vi "TuningPanel.vi"() -> ()   [LabVIEW 2014]
panel:
  in  "Cancel Button":bool
  in  "TCPConRef":refnum<k5>
  in  "Tuning Element":u16(ring) items=["NonlinearPID", "KalmanFilterRegular", "KalmanFilterAltitude", "AttitudeObserver", "HGObserver"]
  in  "OK Button":bool
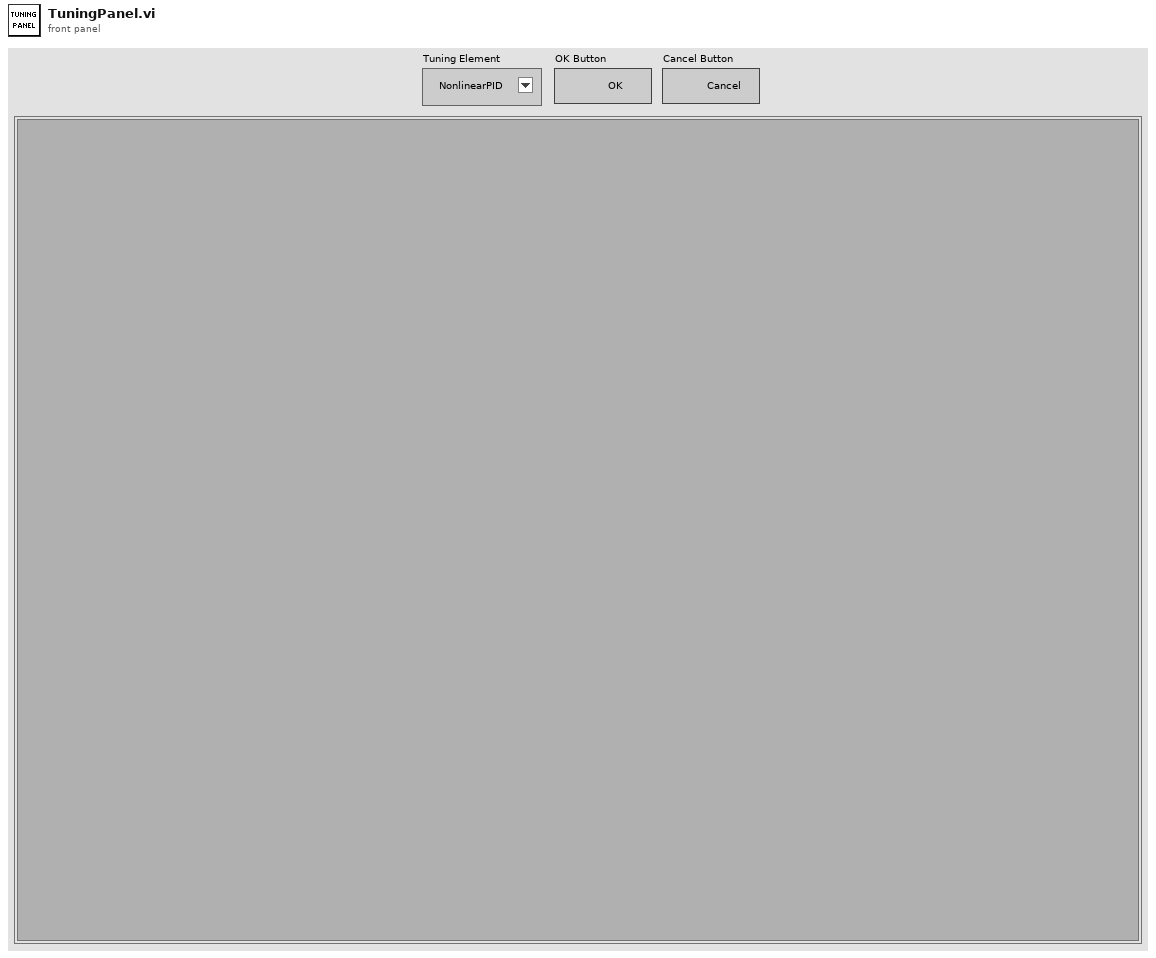
[diagram p1: front panel]
types:
  T1 = enum16{"open", "replace", "create", "open or create", "replace or create", "replace or create with confirmation"}
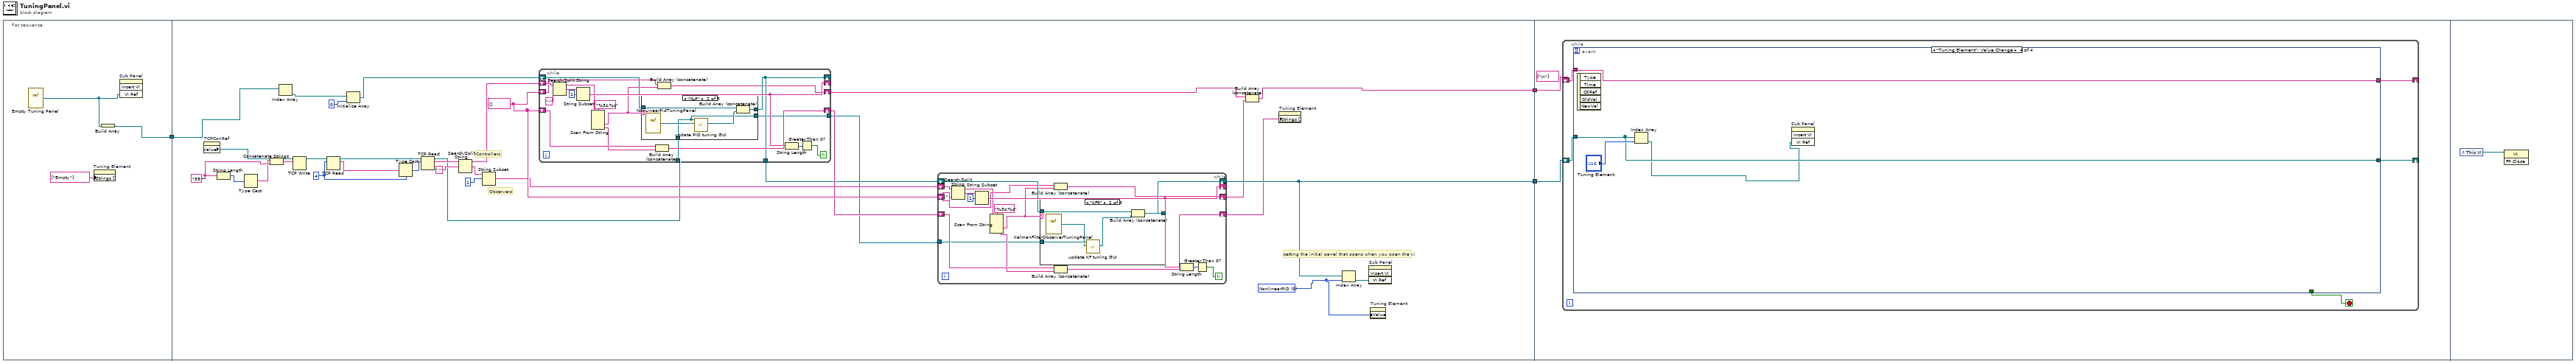
[diagram p0: block diagram]
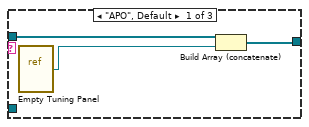
[diagram p2: hidden frame]
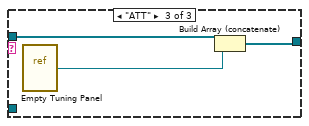
[diagram p3: hidden frame]
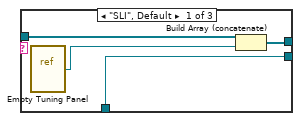
[diagram p4: hidden frame]
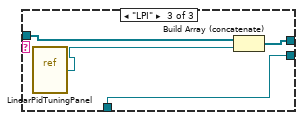
[diagram p5: hidden frame]
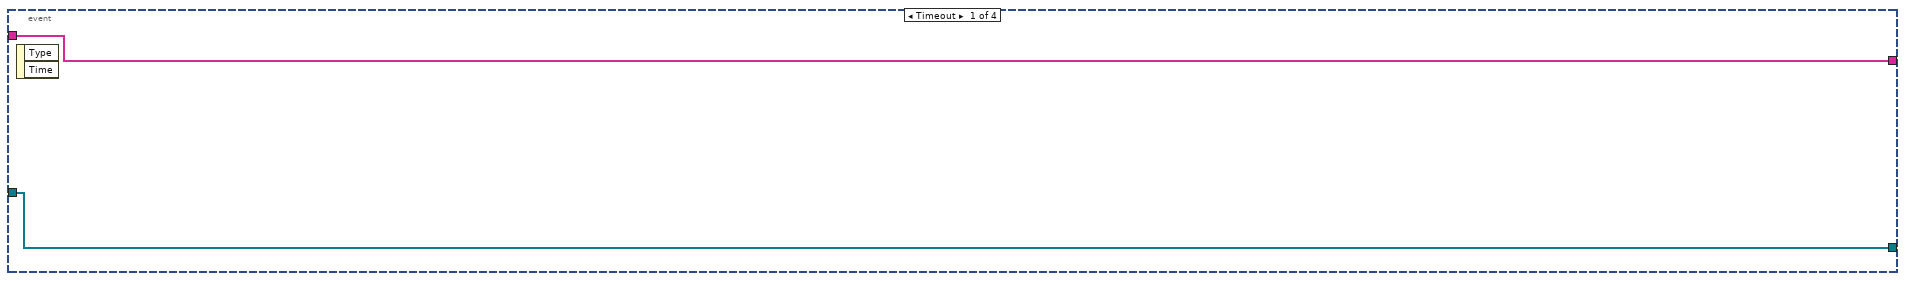
[diagram p6: hidden frame]
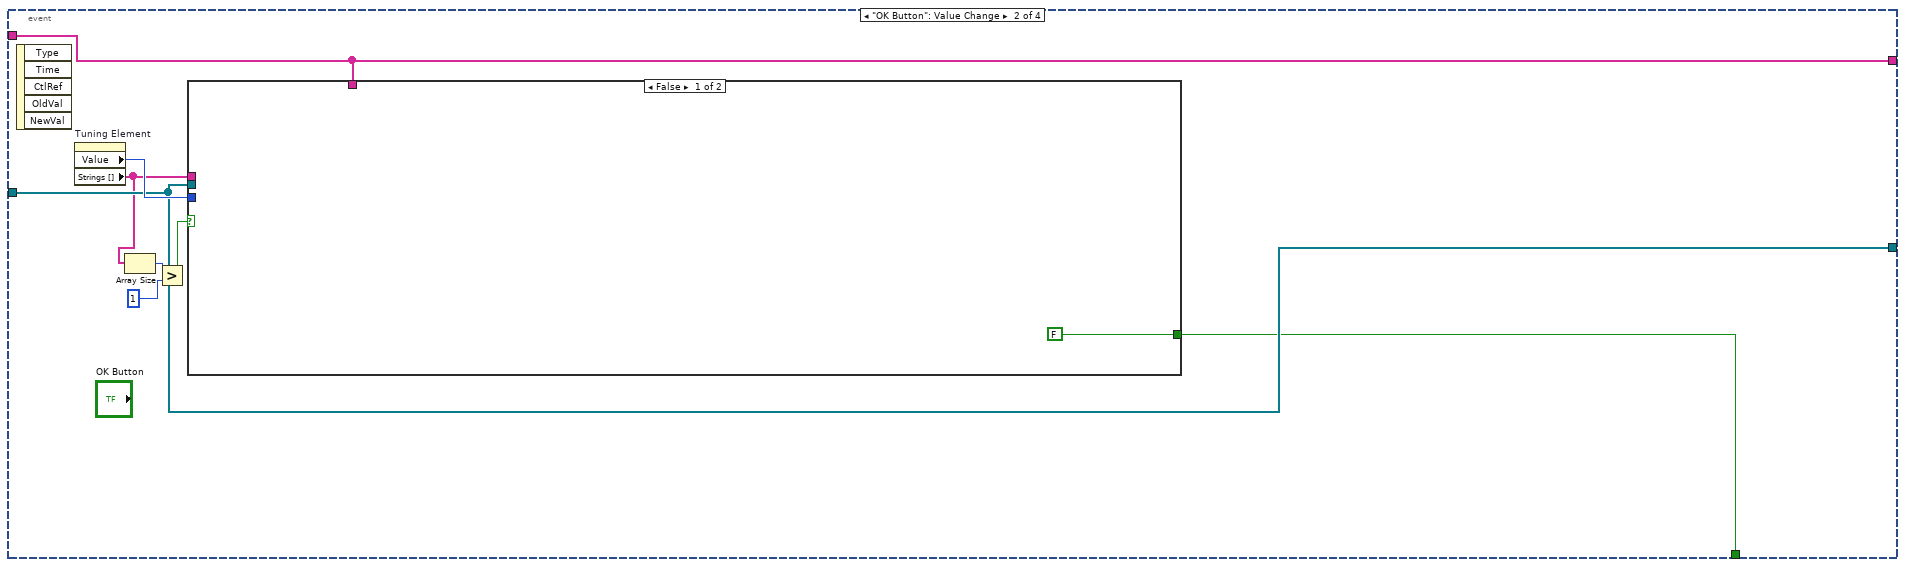
[diagram p7: hidden frame]
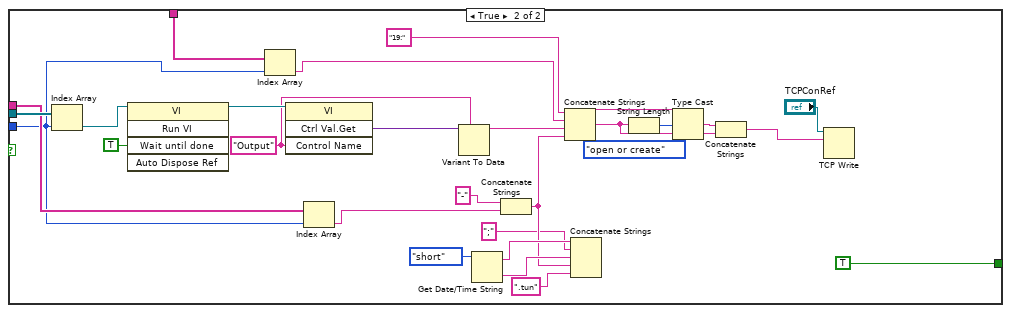
[diagram p8: hidden frame]
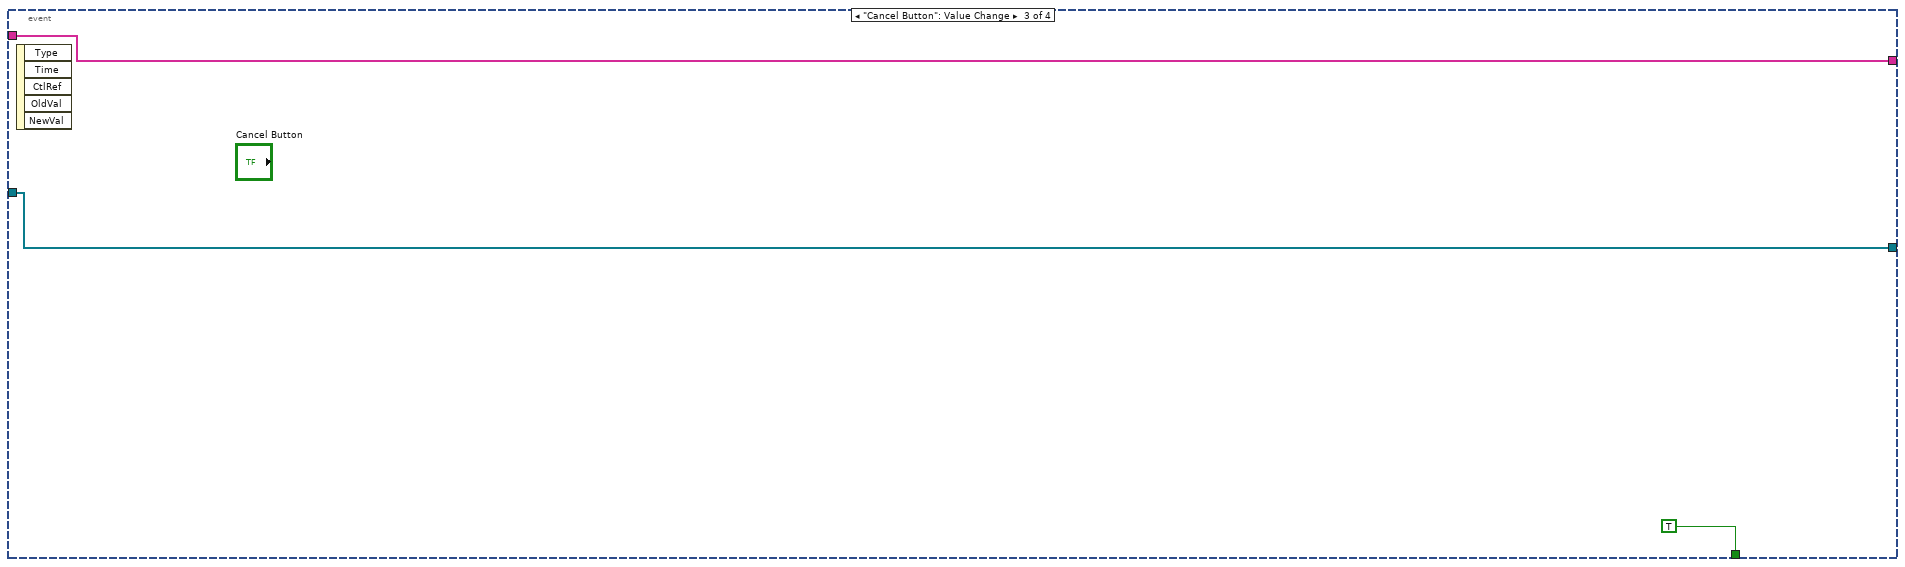
[diagram p9: hidden frame]
diagram:
  n1 = flat-sequence {
    tunnel: [w5] -> w3
    tunnel: [w37] -> w2
    tunnel: [w36] -> w1
    tunnel: w3 -> [w38]
    tunnel: w2 -> [w101]
    tunnel: w1 -> [w100]
    frame #0 {
      n2 = vi-ref "Empty Tuning Panel.vi"() -> (w6:refnum<vi>)
      n3 = property on="Tuning Element" class="Ring (strict)"("Strings []"=string[] ["Empty"]) -> ()  [unwired: 2 in, 2 out]
      n4 = Build Array(w6) -> (w5:refnum<vi>[])
      n5 = invoke on="Sub Panel" class="SubPanel" method="Insert VI"("VI Ref"=w6) -> ()  [unwired: 3 in, 4 out]
    }
    frame #1 {
      w11 = u16 0 items=["NonlinearPID", "KalmanFilterRegular", "KalmanFilterAltitude", "AttitudeObserver", "HGObserver"] ("Tuning Element 2")
      w33 = string[] []
      w19 = 4
      w16 = "38:"
      # "setting the initial panel that opens when you open the vi"
      # "Controllers"
      # "Observers"
      n6 = property on="TCPConRef" class="Ref (strict)"() -> ("Value"=w10:refnum<k5>)  [unwired: 2 in, 2 out]
      n7 = String Length(string=w16) -> (length=w14:i32)
      n8 = Type Cast(x=w14) -> (*(type *) &x=w15:string)  [unwired: 1 in]
      n9 = Concatenate Strings(w15, w16) -> (w17:string)
      n10 = Index Array(array=w38) -> (element=w25:refnum<vi>)  [unwired: 1 in]
      n11 = TCP Write(connection ID=w10, data in=w17) -> (connection ID out=w13:refnum<k5>)  [unwired: 2 in, 2 out]
      n12 = TCP Read(connection ID=w13, bytes to read=w19) -> (connection ID out=w9:refnum<k5>, data out=w18:string)  [unwired: 3 in, 1 out]
      n13 = Initialize Array(w25, 0) -> (w27:refnum<vi>[])
      n14 = Type Cast(type=w19, x=w18) -> (*(type *) &x=w31:i32)
      n15 = TCP Read(connection ID=w9, bytes to read=w31) -> (connection ID out=w8:refnum<k5>, data out=w20:string)  [unwired: 3 in, 1 out]
      n16 = Search/Split String(string=w20, search string/char (-)=",") -> (substring before match=w24:string, match + rest of string=w22:string)  [unwired: 1 in, 1 out]
      n17 = String Subset(string=w22, offset (0)=1) -> (substring=w30:string)  [unwired: 1 in]
      n18 = while {
        shift-right: [w80] -> _
        shift-left: w24 -> [w86]
        shift-right: [w76] -> w29
        shift-left: w33 -> [w75]
        shift-right: [w73] -> _
        shift-left: w27 -> [w74]
        tunnel: [w73] -> w28
        shift-right: [w71] -> w34
        shift-left: w33 -> [w70]
        tunnel: w8 -> [w69]
        tunnel: [w68] -> w7
        stop <- w78 continue-if-true
        n19 = Search/Split String(string=w86, search string/char (-)=";") -> (substring before match=w82:string, match + rest of string=w84:string)  [unwired: 1 in, 1 out]
        n20 = String Subset(string=w84, offset (0)=1) -> (substring=w80:string)  [unwired: 1 in]
        n21 = Scan From String(format string="%3s:%s", input string=w82) -> (output 1=w72:string, output 2=w77:string)  [unwired: 4 in, 3 out]
        n22 = case shown="\"NLP\"" w72 {
          tunnel: w74 -> [w89 w95 w99]
          tunnel: [w88 w94 w98] -> w73
          tunnel: w69 -> [w87 w91 w96]
          tunnel: [w87 w91 w96] -> w68
          frame "SLI", Default {
            n23 = vi-ref "Empty Tuning Panel.vi"() -> (w90:refnum<vi>)
            n24 = Build Array (concatenate)(w89, w90) -> (w88:refnum<vi>[])
          }
          frame "NLP" {
            n25 = vi-ref "NonLinearPidTuningPanel.vi"() -> (w93:refnum<vi>)
            n26 = call "update PID tuning GUI.vi"("reference"=w93, "TCP Network Connection in"=w91) -> ("reference out"=w92:refnum<vi>)  [unwired: 9 in]
            n27 = Build Array (concatenate)(w95, w92) -> (w94:refnum<vi>[])
          }
          frame "LPI" {
            n28 = vi-ref "LinearPidTuningPanel.vi"() -> (w97:refnum<vi>)
            n29 = Build Array (concatenate)(w99, w97) -> (w98:refnum<vi>[])
          }
        }
        n30 = Build Array (concatenate)(w75, w77) -> (w76:string[])
        n31 = Build Array (concatenate)(w70, w72) -> (w71:string[])
        n32 = String Length(string=w80) -> (length=w79:i32)
        n33 = Greater Than 0?(x=w79) -> (x > 0?=w78:bool)
      }
      n34 = while {
        shift-right: [w50] -> _
        shift-left: w30 -> [w56]
        shift-right: [w46] -> w32
        shift-left: w29 -> [w45]
        shift-right: [w43] -> w37
        shift-left: w28 -> [w44]
        shift-right: [w40] -> w35
        shift-left: w33 -> [w42]
        tunnel: w7 -> [w39]
        stop <- w48 continue-if-true
        n35 = Search/Split String(string=w56, search string/char (-)=";") -> (substring before match=w52:string, match + rest of string=w54:string)  [unwired: 1 in, 1 out]
        n36 = String Subset(string=w54, offset (0)=1) -> (substring=w50:string)  [unwired: 1 in]
        n37 = Scan From String(format string="%3s:%s", input string=w52) -> (output 1=w41:string, output 2=w47:string)  [unwired: 4 in, 3 out]
        n38 = case shown="\"KFR\"" w41 {
          tunnel: w44 -> [w58 w64 w66]
          tunnel: [w57 w63 w65] -> w43
          tunnel: w39 -> [_ w62 _]
          frame "APO", Default {
            n39 = vi-ref "Empty Tuning Panel.vi"() -> (w59:refnum<vi>)
            n40 = Build Array (concatenate)(w58, w59) -> (w57:refnum<vi>[])
          }
          frame "KFR" {
            n41 = vi-ref "KalmanFilterObserverTuningPanel.vi"() -> (w61:refnum<vi>)
            n42 = call "update KF tuning GUI.vi"("reference"=w61, "TCP Network Connection in"=w62) -> ("reference out"=w60:refnum<vi>)  [unwired: 9 in]
            n43 = Build Array (concatenate)(w64, w60) -> (w63:refnum<vi>[])
          }
          frame "ATT" {
            n44 = vi-ref "Empty Tuning Panel.vi"() -> (w67:refnum<vi>)
            n45 = Build Array (concatenate)(w66, w67) -> (w65:refnum<vi>[])
          }
        }
        n46 = Build Array (concatenate)(w42, w41) -> (w40:string[])
        n47 = Build Array (concatenate)(w45, w47) -> (w46:string[])
        n48 = String Length(string=w50) -> (length=w49:i32)
        n49 = Greater Than 0?(x=w49) -> (x > 0?=w48:bool)
      }
      n50 = Build Array (concatenate)(w34, w35) -> (w36:string[])
      n51 = property on="Tuning Element" class="Ring (strict)"("Strings []"=w32) -> ()  [unwired: 2 in, 2 out]
      n52 = Index Array(array=w37, index=w11) -> (element=w12:refnum<vi>)
      n53 = invoke on="Sub Panel" class="SubPnl" method="Insert VI"("VI Ref"=w12) -> ()  [unwired: 3 in, 4 out]
      n54 = property on="Tuning Element" class="Ring (strict)"("Value"=w11) -> ()  [unwired: 2 in, 2 out]
    }
    frame #2 {
      (unwired) string[] ["\n"]
      n55 = while {
        shift-right: [w104] -> _
        shift-left: w101 -> [w106]
        shift-right: [w103] -> _
        shift-left: w100 -> [w102]
        stop <- w105 stop-if-true
        n56 = event shown="[3] \"Tuning Element\": Value Change" {
          selector: _ -> [_ _ _ _]
          dyn-events: _ -> [_ _ _ _]
          timeout: _ -> [_ _ _ _]
          tunnel: w106 -> [w108 w115 w145 w149]
          tunnel: [_ w109 TRUE _] -> w105
          tunnel: [w108 w115 w145 w149] -> w104
          tunnel: [w107 w110 w144 w148] -> w103
          tunnel: w102 -> [w107 w110 w144 w148]
          event Timeout {
            n57 = event-data() -> ()  [unwired: 1 in, 2 out]
          }
          event "OK Button": Value Change {
            n58 = event-data() -> ()  [unwired: 1 in, 5 out]
            n59 = property on="Tuning Element" class="Ring (strict)"() -> ("Value"=w116:u16, "Strings []"=w114:string[])  [unwired: 2 in, 2 out]
            n60 = Array Size(array=w114) -> (size(s)=w113:i32)
            n61 = Greater?(x=w113, y=1) -> (0:w111:bool)
            n62 = case shown="False" w111 {
              tunnel: w116 -> [_ w128]
              tunnel: w115 -> [_ w131]
              tunnel: w114 -> [_ w130]
              tunnel: w110 -> [_ w129]
              tunnel: [FALSE TRUE] -> w109
              frame False {
              }
              frame True {
                (unwired) T1."open or create" ("operation (0:open)")
                w139 = "Output" ("Control Name")
                n63 = Index Array(array=w131, index=w128) -> (element=w143:refnum<vi>)
                n64 = invoke class="VI" method="Run VI"(reference=w143, "Wait until done"=TRUE ("Wait Until Done")) -> (reference out=w142:refnum<vi>)  [unwired: 3 in, 4 out]
                n65 = Index Array(array=w129, index=w128) -> (element=w127:string)
                n66 = invoke class="VI" method="Ctrl Val.Get"(reference=w142, "Control Name"=w139) -> ("Get Control Value Variant"=w140:variant)  [unwired: 2 in, 3 out]
                n67 = Index Array(array=w130, index=w128) -> (element=w132:string)
                n68 = Variant To Data(type=w139, Variant=w140) -> (data=w138:string)  [unwired: 1 in, 1 out]
                n69 = Get Date/Time String(date format (0)=enum16{"short", "long", "abbreviated"}."short") -> (date string=w124:string, time string=w123:string)  [unwired: 2 in]
                n70 = Concatenate Strings("-", w132) -> (w120:string)
                n71 = Concatenate Strings("19:" ("string"), w127, w138, w120) -> (w118:string)
                n72 = Concatenate Strings(w124, ";", w123, w120, ".tun") -> ()  [unwired: 1 out]
                n73 = String Length(string=w118) -> (length=w137:i32)
                n74 = Type Cast(type=w118, x=w137) -> (*(type *) &x=w136:string)
                n75 = Concatenate Strings(w136, w118) -> (w135:string)
                n76 = TCP Write(connection ID="TCPConRef", data in=w135) -> ()  [unwired: 2 in, 3 out]
              }
            }
          }
          event "Cancel Button": Value Change {
            n77 = event-data() -> ()  [unwired: 1 in, 5 out]
          }
          event "Tuning Element": Value Change {
            n78 = event-data() -> ()  [unwired: 1 in, 5 out]
            n79 = Index Array(array=w149, index="Tuning Element") -> (element=w147:refnum<vi>)
            n80 = invoke on="Sub Panel" class="SubPnl" method="Insert VI"("VI Ref"=w147) -> ()  [unwired: 3 in, 4 out]
          }
        }
      }
    }
    frame #3 {
      n81 = control-ref of="This VI"() -> (w151:refnum<vi>)
      n82 = invoke class="VI" method="FP.Close"(reference=w151) -> ()  [unwired: 2 in, 3 out]
    }
  }
